vi "test2.vi"() -> ()   [LabVIEW 2012]
uses:
  configlib.lvlib
  Configuration File Definition.ctl
  File Options.ctl
panel:
  out "data value":T1={"dirty"=FALSE, "path"=path "", "Fileopts"={"Name/Value delimiter (\"=\")"="=", "Comment delimiter (\";\")"=";"}, "Section Lookup"=variant, "Key Lookup"=variant, "Raw File"=[]}
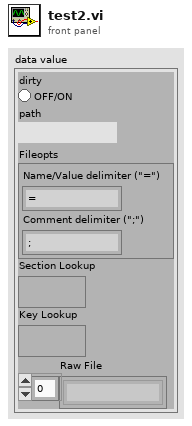
[diagram p1: front panel]
types:
  T1 = typedef "configlib.lvlib/Configuration File Definition.ctl" = cluster{"dirty":bool, "path":path, "Fileopts":T2, "Section Lookup":variant, "Key Lookup":variant, "Raw File":string[]}
  T2 = typedef "configlib.lvlib/File Options.ctl" = cluster{"Name/Value delimiter (\"=\")":string, "Comment delimiter (\";\")":string}
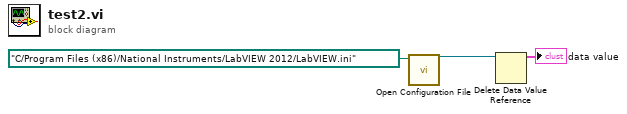
[diagram p0: block diagram]
diagram:
  n1 = call "Open Configuration File.vi"("configuration file path"=path "C:/Program Files (x86)/National Instruments/LabVIEW 2012/LabVIEW.ini") -> ("Configuration Reference"=w3:refnum<data-value>)  [unwired: 8 in, 2 out]
  n2 = Delete Data Value Reference(data value reference=w3) -> (data value=→"data value":T1)  [unwired: 1 in, 1 out]
